vi "Create RPC Method from Template.vi"(7 "New method names":string[](array[string]), 8 "error in (no error)":errorcluster, 11 "Server class in":refnum<vi>) -> (0 "error out":errorcluster, 3 "Server class out":refnum<vi>)   [LabVIEW 2019, in "gRPC Scripting Tools.lvlib"]
uses:
  gRPC Scripting Tools.lvlib
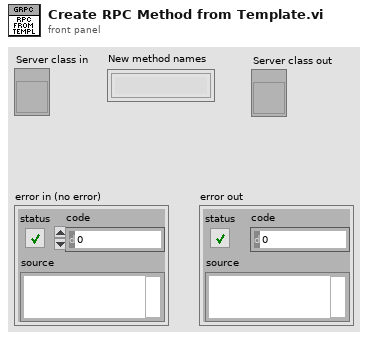
[diagram p1: front panel]
types:
  T1 = enum32{"invalid VI type", "Standard VI", "Control VI", "Global VI", "Polymorphic VI", "Configuration VI", "SubSystem", "Facade VI", "Method VI"}
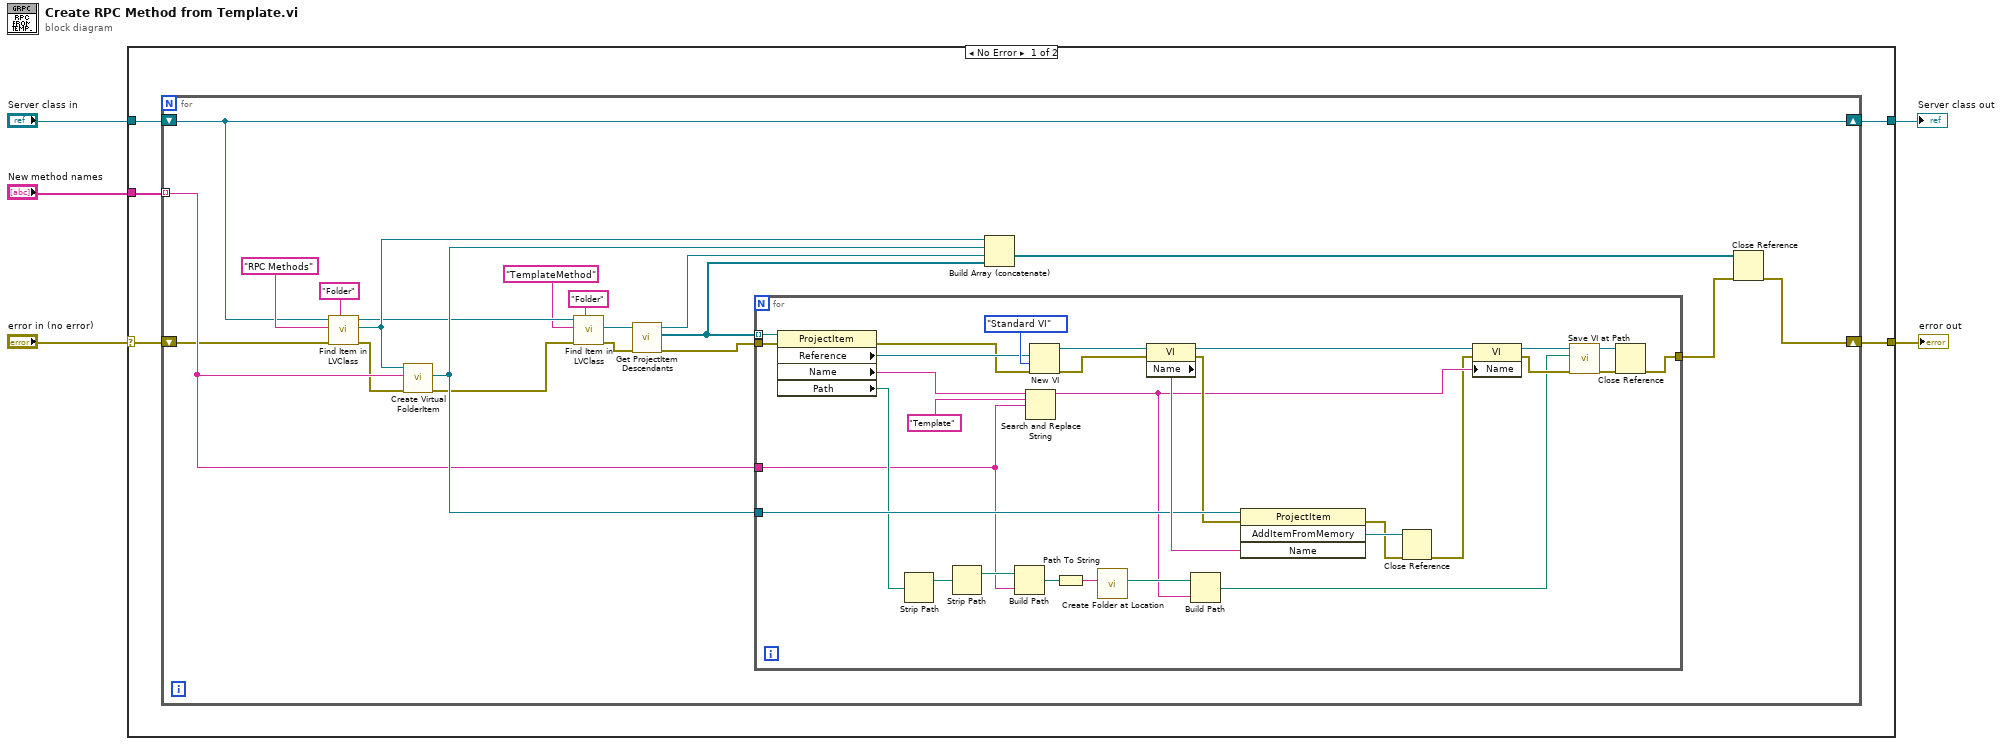
[diagram p0: block diagram]
diagram:
  n1 = case shown="No Error" "error in (no error)" {
    selector: "error in (no error)" -> [w8 w62]
    tunnel: "New method names" -> [w10 _]
    tunnel: [w9 w62] -> w5
    tunnel: "Server class in" -> [w7 w61]
    tunnel: [w6 w61] -> w2
    frame No Error {
      n2 = for {
        tunnel: w10 -> [w28] mode=indexing
        shift-right: [w25] -> w9
        shift-left: w8 -> [w12]
        shift-right: [w11] -> w6
        shift-left: w7 -> [w11]
        n3 = call "Find Item in LVClass.vi"("Item Type"="Folder", "error in (no error)"=w12, "Item Name"="RPC Methods", "Class Item in"=w11) -> ("error out"=w26:errorcluster, "Project Item (Class Item)"=w29:refnum<vi>, "Class Item out"=w19:refnum<vi>)  [unwired: 4 in, 1 out]
        n4 = call "Create Virtual FolderItem.vi"("error in (no error)"=w26, "Folder Name"=w28, "ProjectItem in"=w29) -> ("error out"=w27:errorcluster, "FolderItem reference out"=w30:refnum<vi>)  [unwired: 6 in, 1 out]
        n5 = call "Find Item in LVClass.vi"("Item Type"="Folder", "error in (no error)"=w27, "Item Name"="TemplateMethod", "Class Item in"=w19) -> ("error out"=w15:errorcluster, "Project Item (Class Item)"=w16:refnum<vi>)  [unwired: 4 in, 2 out]
        n6 = call "Get ProjectItem Descendants.vi"("error in (no error)"=w15, "ProjectItem in"=w16) -> ("error out"=w20:errorcluster, "All Descendents"=w21:refnum<vi>[], "ProjectItem out"=w22:refnum<vi>)  [unwired: 7 in]
        n7 = for {
          tunnel: w21 -> [w60] mode=indexing
          tunnel: w30 -> [w53]
          tunnel: [w36] -> w23
          tunnel: w20 -> [w31]
          tunnel: w28 -> [w41]
          n8 = property class="ProjectItem"(reference=w60, error in=w31) -> (error out=w51:errorcluster, "Reference"=w54:refnum<vi>, "Name"=w59:string, "Path"=w46:path)  [unwired: 1 out]
          n9 = Strip Path(path=w46) -> (stripped path=w45:path)  [unwired: 1 out]
          n10 = Strip Path(path=w45) -> (stripped path=w44:path)  [unwired: 1 out]
          n11 = Build Path(base path=w44, name or relative path=w41) -> (appended path=w43:path)
          n12 = Search and Replace String(input string=w59, search string="Template", replace string=w41) -> (result string=w39:string)  [unwired: 5 in, 3 out]
          n13 = New VI(8:w51, 9:T1."Standard VI" ("vi type (standard vi)"), 10:w54) -> (0:w50:errorcluster, 3:w56:refnum<vi>)  [unwired: 1 in, 3 out]
          n14 = Path To String(path=w43) -> (string=w42:string)
          n15 = call "Create Folder at Location.vi"("Path"=w42) -> ("Full path out"=w40:path)  [unwired: 9 in, 1 out]
          n16 = property class="VI"(reference=w56, error in=w50) -> (reference out=w52:refnum<vi>, error out=w49:errorcluster, "Name"=w57:string)
          n17 = Build Path(base path=w40, name or relative path=w39) -> (appended path=w38:path)
          n18 = invoke class="ProjectItem" method="AddItemFromMemory"(reference=w53, error in=w49, "Name"=w57) -> (error out=w33:errorcluster, "AddItemFromMemory"=w34:refnum<vi>)  [unwired: 1 in, 2 out]
          n19 = Close Reference(reference=w34, error in (no error)=w33) -> (error out=w32:errorcluster)
          n20 = property class="VI"(reference=w52, error in=w32, "Name"=w39) -> (reference out=w48:refnum<vi>, error out=w47:errorcluster)
          n21 = call "Save VI at Path.vi"("error in (no error)"=w47, "Path"=w38, "VI in"=w48) -> ("error out"=w37:errorcluster, "VI out"=w35:refnum<vi>)  [unwired: 6 in, 1 out]
          n22 = Close Reference(reference=w35, error in (no error)=w37) -> (error out=w36:errorcluster)
        }
        n23 = Build Array (concatenate)(w29, w30, w22, w21) -> (w24:refnum<vi>[])
        n24 = Close Reference(reference=w24, error in (no error)=w23) -> (error out=w25:errorcluster)
      }
    }
    frame Error {
    }
  }
  "error out" <- w5
  "Server class out" <- w2
